vi "Send to ROS (SubVI).vi"(6 "frequency":dbl, 7 "ROS IP":string="192.168.0.100", 8 "Good signal?":dbl, 9 "dt 3":dbl, 10 "dt2":dbl, 11 "dt 1":dbl) -> (0 "error out":errorcluster)   [LabVIEW 2012]
uses:
  <vilib>/Clearpath Robotics/ROS Toolkit/ros_toolkit.lvlib
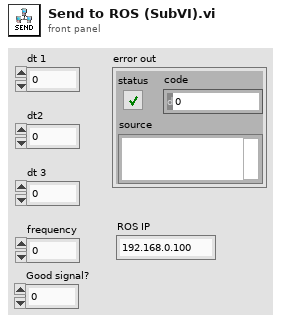
[diagram p1: front panel]
types:
  T1 = cluster{"linear":cluster{"x":dbl, "y":dbl, "z":dbl}, "angular":cluster{"x":dbl, "y":dbl, "z":dbl}}
  T2 = cluster{"connection ID out":refnum<k5>, "Data Buffer":string}
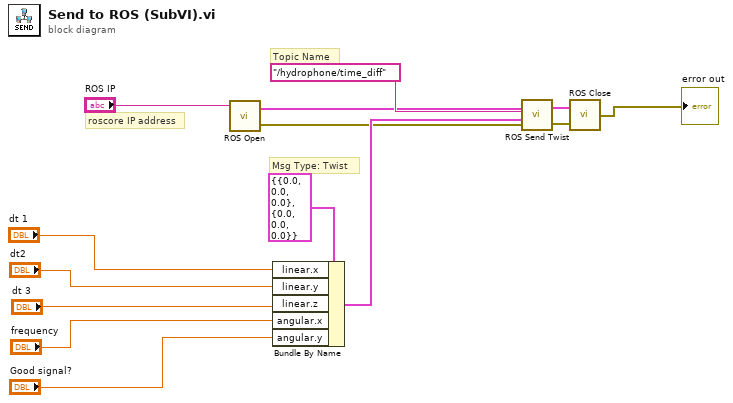
[diagram p0: block diagram]
diagram:
  # "roscore IP address"
  # "Topic Name"
  # "Msg Type: Twist"
  n1 = call <vilib>:"ROS Open.vi"("bridge IP"="ROS IP") -> ("error out"=w7:errorcluster, "ROS link"=w6:T2)  [unwired: 2 in]
  n2 = Bundle By Name(cluster=T1 {"linear"={"x"=0.0, "y"=0.0, "z"=0.0}, "angular"={"x"=0.0, "y"=0.0, "z"=0.0}} ("twist"), "linear.x"="dt 1", "linear.y"="dt2", "linear.z"="dt 3", "angular.x"="frequency", "angular.y"="Good signal?") -> (w10:T1)
  n3 = call <vilib>:"ROS Send Twist.vi"("error in"=w7, "twist"=w10, "receiver (/cmd_vel)"="/hydrophone/time_diff" ("Command Topic"), "ROS link In"=w6) -> ("error out"=w5:errorcluster, "ROS link Out"=w4:T2)
  n4 = call <vilib>:"ROS Close.vi"("error in"=w5, "ROS link"=w4) -> ("error out"=→"error out":errorcluster)
